vi "BlinkSdkExample.vi"   [LabVIEW 2010]
uses:
  ImageGen.dll
  Program Files/Meadowlark Optics/Blink 1920 HDMI/SDK/Blink_C_wrapper.dll
panel:
  # "Demonstrates how to load images to the SLM by looping though 2 images 5 times each"
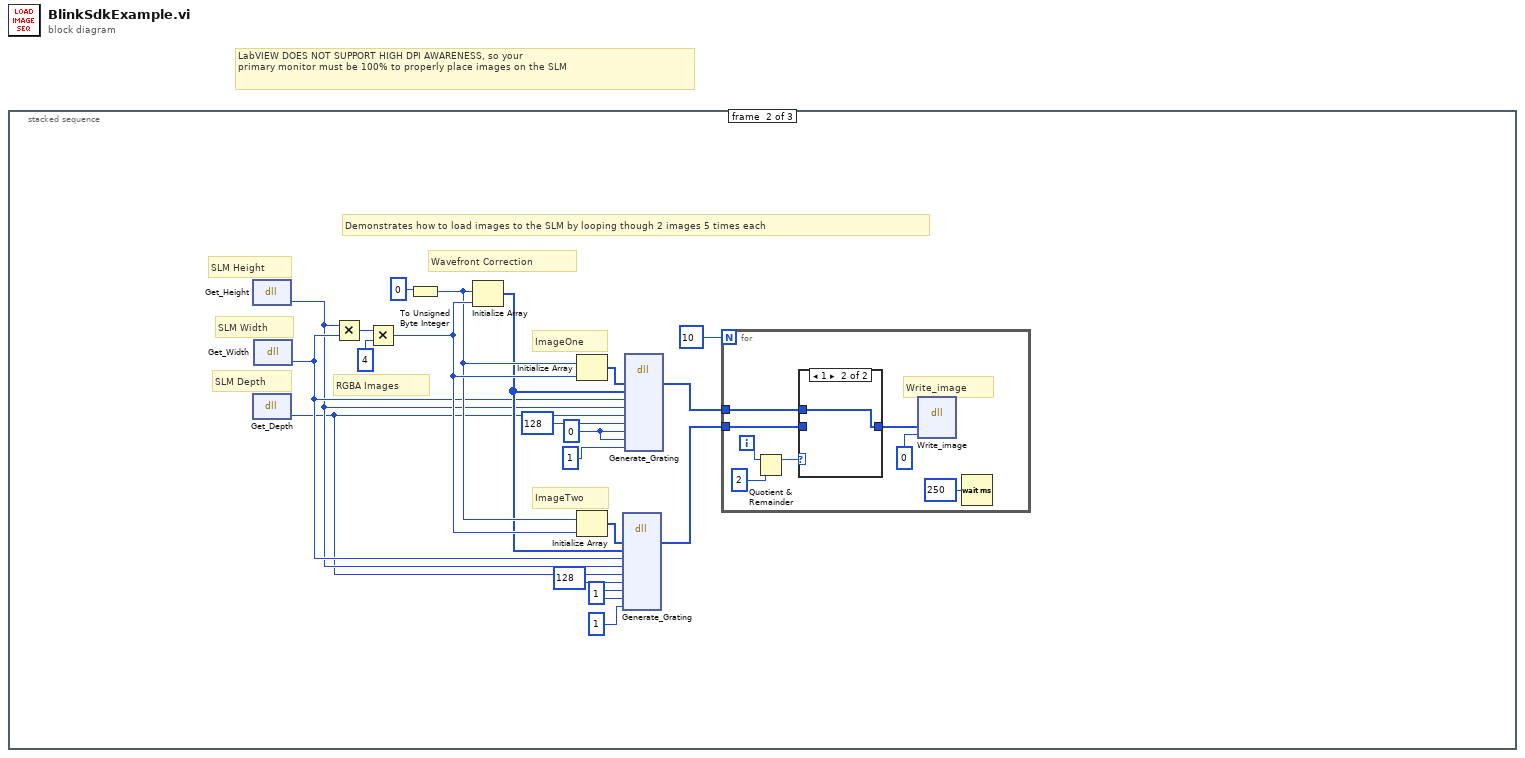
[diagram p0: block diagram]
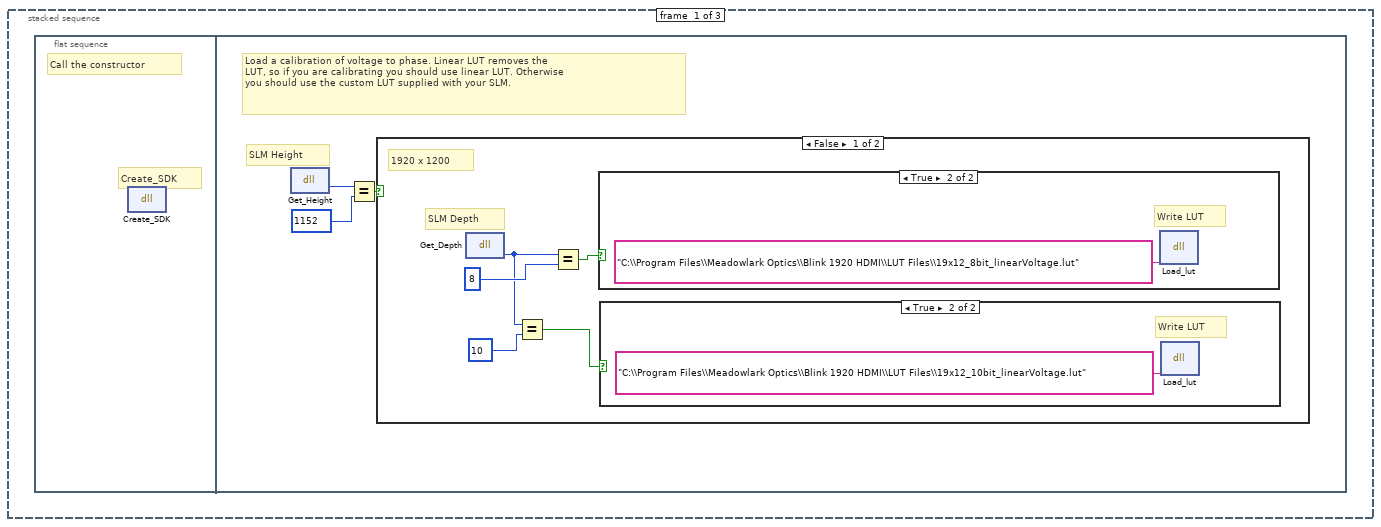
[diagram p2: hidden frame]
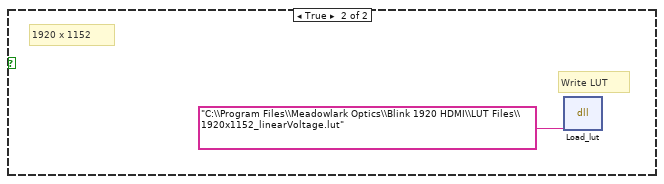
[diagram p5: hidden frame]
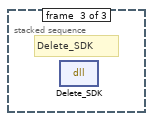
[diagram p7: hidden frame]
diagram:
  # "LabVIEW DOES NOT SUPPORT HIGH DPI AWARENESS, so your \nprimary monitor must be 100% to properly place images on the SLM"
  n1 = stacked-sequence {
    frame #0 {
      n2 = flat-sequence {
        frame #0 {
          # "Call the constructor"
          # "Create_SDK"
          n3 = dll-call lib="C:/Program Files/Meadowlark Optics/Blink 1920 HDMI/SDK/Blink_C_wrapper.dll" fn="Create_SDK"() -> ()  [unwired: 4 in, 2 out]
        }
        frame #1 {
          # "SLM Height"
          # "Load a calibration of voltage to phase. Linear LUT removes the \nLUT, so if you are calibrating you should use linear LUT. Otherwise \nyou should use the custom LUT supplied with your SLM."
          n4 = dll-call lib="C:/Program Files/Meadowlark Optics/Blink 1920 HDMI/SDK/Blink_C_wrapper.dll" fn="Get_Height"() -> ("return type"=w1:i32)  [unwired: 3 in, 2 out]
          n5 = Equal?(x=w1, y=1152) -> (x = y?=w3:bool)
          n6 = case shown="False" w3 {
            frame False {
              # "1920 x 1200"
              # "SLM Depth"
              n7 = dll-call lib="C:/Program Files/Meadowlark Optics/Blink 1920 HDMI/SDK/Blink_C_wrapper.dll" fn="Get_Depth"() -> ("return type"=w7:i32)  [unwired: 3 in, 2 out]
              n8 = Equal?(x=w7, y=10) -> (x = y?=w5:bool)
              n9 = Equal?(x=w7, y=8) -> (x = y?=w4:bool)
              n10 = case shown="True" w4 {
                frame False {
                }
                frame True {
                  # "Write LUT"
                  n11 = dll-call lib="C:/Program Files/Meadowlark Optics/Blink 1920 HDMI/SDK/Blink_C_wrapper.dll" fn="Load_lut"("Path"="C:\\Program Files\\Meadowlark Optics\\Blink 1920 HDMI\\LUT Files\\19x12_8bit_linearVoltage.lut") -> ()  [unwired: 5 in, 2 out]
                }
              }
              n12 = case shown="True" w5 {
                frame False {
                }
                frame True {
                  # "Write LUT"
                  n13 = dll-call lib="C:/Program Files/Meadowlark Optics/Blink 1920 HDMI/SDK/Blink_C_wrapper.dll" fn="Load_lut"("Path"="C:\\Program Files\\Meadowlark Optics\\Blink 1920 HDMI\\LUT Files\\19x12_10bit_linearVoltage.lut") -> ()  [unwired: 5 in, 2 out]
                }
              }
            }
            frame True {
              # "1920 x 1152"
              # "Write LUT"
              n14 = dll-call lib="C:/Program Files/Meadowlark Optics/Blink 1920 HDMI/SDK/Blink_C_wrapper.dll" fn="Load_lut"("Path"="C:\\Program Files\\Meadowlark Optics\\Blink 1920 HDMI\\LUT Files\\1920x1152_linearVoltage.lut") -> ()  [unwired: 5 in, 2 out]
            }
          }
        }
      }
    }
    frame #1 {
      w26 = 1
      w28 = 0
      # "RGBA Images"
      # "SLM Depth"
      # "SLM Width"
      # "SLM Height"
      # "ImageTwo"
      # "ImageOne"
      # "Wavefront Correction"
      # "Demonstrates how to load images to the SLM by looping though 2 images 5 times each"
      n15 = dll-call lib="C:/Program Files/Meadowlark Optics/Blink 1920 HDMI/SDK/Blink_C_wrapper.dll" fn="Get_Height"() -> ("return type"=w17:i32)  [unwired: 3 in, 2 out]
      n16 = dll-call lib="C:/Program Files/Meadowlark Optics/Blink 1920 HDMI/SDK/Blink_C_wrapper.dll" fn="Get_Depth"() -> ("return type"=w16:i32)  [unwired: 3 in, 2 out]
      n17 = dll-call lib="C:/Program Files/Meadowlark Optics/Blink 1920 HDMI/SDK/Blink_C_wrapper.dll" fn="Get_Width"() -> ("return type"=w18:i32)  [unwired: 3 in, 2 out]
      n18 = Multiply(x=w17, y=w18) -> (x*y=w24:i32)
      n19 = Multiply(x=w24, y=4) -> (x*y=w22:i32)
      n20 = To Unsigned Byte Integer(number=0) -> (unsigned 8bit integer=w20:u8)
      n21 = Initialize Array(w20, w22) -> (w19:u8[])
      n22 = Initialize Array(w20, w22) -> (w30:u8[])
      n23 = Initialize Array(w20, w22) -> (w27:u8[])
      n24 = dll-call lib="C:/Meadowlark/Repos-git/MeadowlarkBison/BlinkSdkExample/ImageGen.dll" fn="Generate_Grating"("Array"=w27, "WFC"=w19, "Width"=w18, "Height"=w17, "Depth"=w16, "Period"=128, "Increasing"=w26, "Horizontal"=w26, "RGB"=1) -> ("Array"=w14:u8[])  [unwired: 12 in, 2 out]
      n25 = dll-call lib="C:/Meadowlark/Repos-git/MeadowlarkBison/BlinkSdkExample/ImageGen.dll" fn="Generate_Grating"("Array"=w30, "WFC"=w19, "Width"=w18, "Height"=w17, "Depth"=w16, "Period"=128, "Increasing"=w28, "Horizontal"=w28, "RGB"=1) -> ("Array"=w15:u8[])  [unwired: 12 in, 2 out]
      n26 = for {
        N: 10 -> [_]
        tunnel: w15 -> [w34]
        tunnel: w14 -> [w33]
        i -> [w37]
        # "Write_image"
        n27 = Quotient & Remainder(x=w37, y=2) -> (x-y*floor(x/y)=w36:i32)  [unwired: 1 out]
        n28 = case shown="1" w36 {
          tunnel: w34 -> [_ w41]
          tunnel: w33 -> [w40 _]
          tunnel: [w40 w41] -> w32
          frame 0, Default {
          }
          frame 1 {
          }
        }
        n29 = dll-call lib="C:/Program Files/Meadowlark Optics/Blink 1920 HDMI/SDK/Blink_C_wrapper.dll" fn="Write_image"("image_data"=w32, "isEightBit"=0) -> ()  [unwired: 6 in, 2 out]
        n30 = Wait (ms)(milliseconds to wait=u32 250) -> ()  [unwired: 1 out]
      }
    }
    frame #2 {
      # "Delete_SDK"
      n31 = dll-call lib="C:/Program Files/Meadowlark Optics/Blink 1920 HDMI/SDK/Blink_C_wrapper.dll" fn="Delete_SDK"() -> ()  [unwired: 4 in, 2 out]
    }
  }
